vi "SelectValueDC.vi"(8 "error in (no error)":errorcluster, 9 "Table Row Name":string, 10 "Unique Object Identifier":string, 11 "DataCollector in":refnum<class "DataCollector.lvclass">) -> (0 "error out":errorcluster, 2 "Value":string, 3 "DataCollector out":refnum<class "DataCollector.lvclass">)   [LabVIEW 2017, in "DataCollector.lvclass"]
uses:
  DataCollector.lvclass
  <vilib>/drjdpowell/SQLite Library/SQL Statement/SQL Statement.lvclass
  <vilib>/drjdpowell/SQLite Library/SQL Connection/Connection.lvclass
panel:
  out "Dezimal-Integer-String":string
  out "concatenated string":string
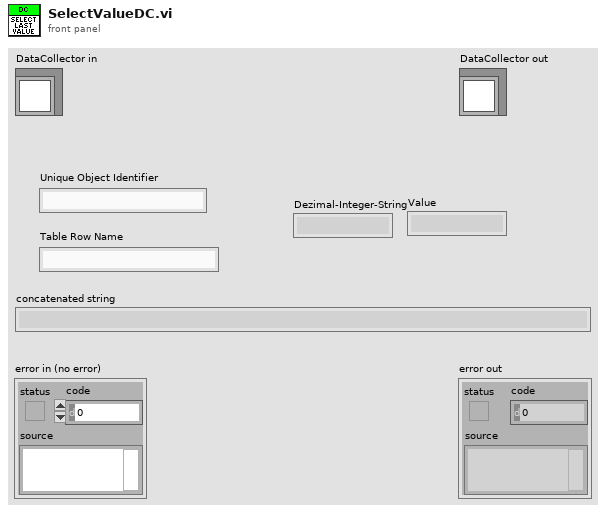
[diagram p1: front panel]
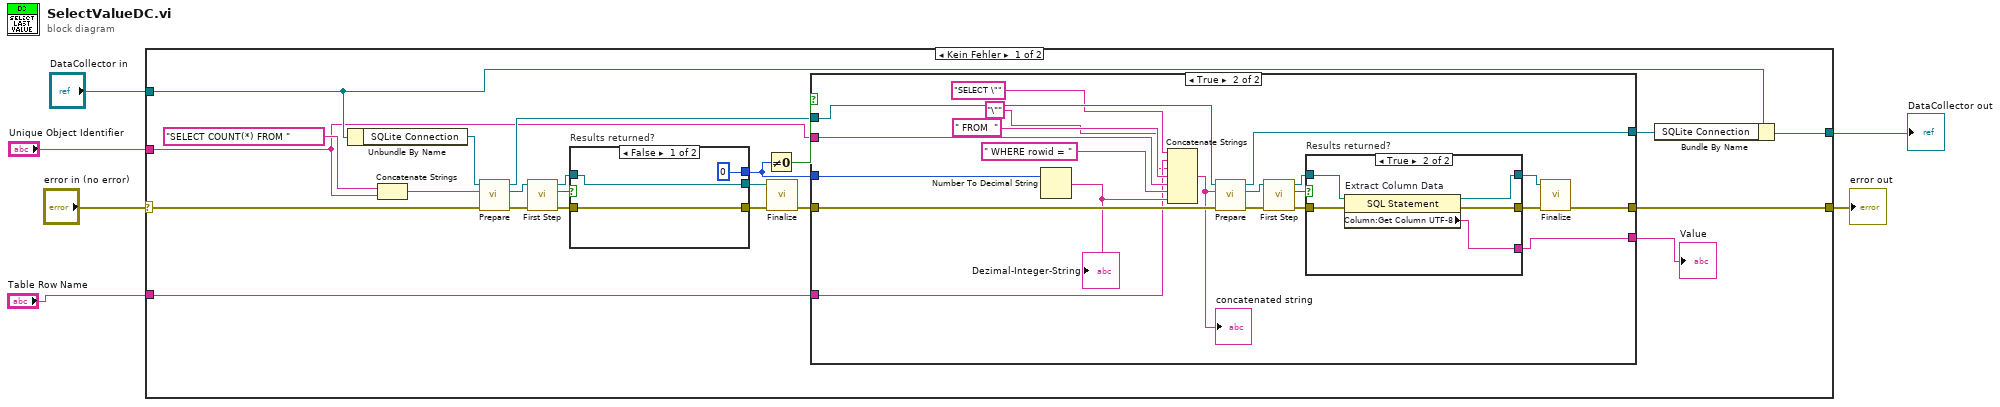
[diagram p0: block diagram]
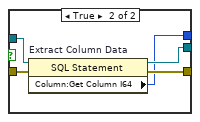
[diagram p2: hidden frame]
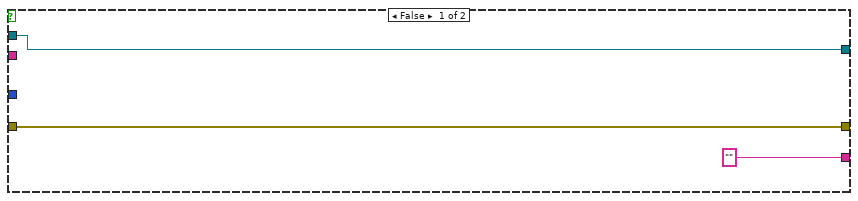
[diagram p3: hidden frame]
diagram:
  n1 = case shown="Kein Fehler" "error in (no error)" {
    selector: "error in (no error)" -> [w12 w69]
    tunnel: [w26 w69] -> w4
    tunnel: [w27 w68] -> w5
    tunnel: "DataCollector in" -> [w28 w68]
    tunnel: "Unique Object Identifier" -> [w10 _]
    tunnel: "Table Row Name" -> [w8 _]
    frame No Error {
      n2 = Unbundle By Name(w28) -> ("SQLite Connection"=w16:refnum<class "Connection.lvclass">)
      n3 = Concatenate Strings("SELECT COUNT(*) FROM " ("String"), w10) -> (w9:string)
      n4 = call <vilib>:"Prepare.vi"("error in (no error)"=w12, "SQL"=w9, "SQLite Connection in"=w16) -> ("error out"=w17:errorcluster, "SQL Statement"=w18:refnum<class "SQL Statement.lvclass">, "SQLite Connection"=w15:refnum<class "Connection.lvclass">)  [unwired: 4 in, 2 out]
      n5 = call <vilib>:"First Step.vi"("error in (no error)"=w17, "SQL Statement in"=w18) -> ("error out"=w19:errorcluster, "Row returned"=w21:bool, "SQL Statement"=w20:refnum<class "SQL Statement.lvclass">)  [unwired: 7 in]
      n6 = case "Results returned?" shown="False" w21 {
        tunnel: [w31 w33] -> w23
        tunnel: [w30 w34] -> w22
        tunnel: w20 -> [w31 w36]
        tunnel: w19 -> [w30 w35]
        tunnel: [i64 0 ("Column:Get Column I64") w32] -> w14
        frame False {
        }
        frame True {
          n7 = property on="Extract Column Data" class="SQL Statement"(reference=w36, error in=w35) -> (reference out=w33:refnum<class "SQL Statement.lvclass">, error out=w34:errorcluster, "Column:Get Column I64"=w32:i64)
        }
      }
      n8 = Not Equal To 0?(x=w14) -> (x != 0?=w24:bool)
      n9 = call <vilib>:"Finalize.vi"("error in (no error)"=w22, "SQL Statement in"=w23) -> ("error out"=w13:errorcluster)  [unwired: 9 in]
      n10 = case shown="True" w24 {
        tunnel: [w39 w60] -> w26
        tunnel: w15 -> [w38 w57]
        tunnel: [w38 w56] -> w25
        tunnel: w13 -> [w39 w51]
        tunnel: w14 -> [_ w49]
        tunnel: w10 -> [_ w46]
        tunnel: w8 -> [_ w42]
        tunnel: ["" ("Value") w40] -> w7
        frame False {
        }
        frame True {
          n11 = Number To Decimal String(number=w49) -> (decimal integer string=w43:string)  [unwired: 1 in]
          "Dezimal-Integer-String" <- w43
          n12 = Concatenate Strings("SELECT \"" ("string"), w42, "\"" ("string"), " FROM  " ("string"), w46, " WHERE rowid = " ("string"), w43) -> (w45:string)
          "concatenated string" <- w45
          n13 = call <vilib>:"Prepare.vi"("error in (no error)"=w51, "SQL"=w45, "SQLite Connection in"=w57) -> ("error out"=w59:errorcluster, "SQL Statement"=w58:refnum<class "SQL Statement.lvclass">, "SQLite Connection"=w56:refnum<class "Connection.lvclass">)  [unwired: 4 in, 2 out]
          n14 = call <vilib>:"First Step.vi"("error in (no error)"=w59, "SQL Statement in"=w58) -> ("error out"=w55:errorcluster, "Row returned"=w53:bool, "SQL Statement"=w54:refnum<class "SQL Statement.lvclass">)  [unwired: 7 in]
          n15 = case "Results returned?" shown="True" w53 {
            tunnel: [w62 w64] -> w50
            tunnel: [w61 w65] -> w52
            tunnel: w54 -> [w62 w67]
            tunnel: w55 -> [w61 w66]
            tunnel: [_ w63] -> w40
            frame False {
            }
            frame True {
              n16 = property on="Extract Column Data" class="SQL Statement"(reference=w67, error in=w66) -> (reference out=w64:refnum<class "SQL Statement.lvclass">, error out=w65:errorcluster, "Column:Get Column UTF-8"=w63:string)
            }
          }
          n17 = call <vilib>:"Finalize.vi"("error in (no error)"=w52, "SQL Statement in"=w50) -> ("error out"=w60:errorcluster)  [unwired: 9 in]
        }
      }
      "Value" <- w7
      n18 = Bundle By Name(cluster=w28, "SQLite Connection"=w25) -> (w27:refnum<class "DataCollector.lvclass">)
    }
    frame Error {
    }
  }
  "error out" <- w4
  "DataCollector out" <- w5
